vi "Min_Max_Amp (SubVI).vi"(11 "waveform":waveform(dbl)) -> (1 "AMP.":dbl, 2 "MN":dbl, 3 "MX":dbl)   [LabVIEW 2017]
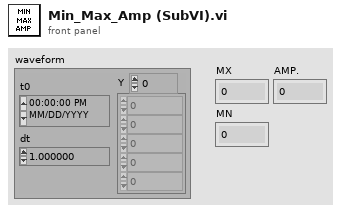
[diagram p1: front panel]
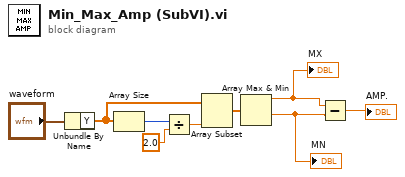
[diagram p0: block diagram]
diagram:
  n1 = Unbundle By Name("waveform") -> ("Y"=w8:dbl[])
  n2 = Array Size(array=w8) -> (size(s)=w6:i32)
  n3 = Divide(x=w6, y=2.0 ("Min Value")) -> (x/y=w5:dbl)
  n4 = Array Subset(array=w8, length=w5) -> (w9:dbl[])  [unwired: 1 in]
  n5 = Array Max & Min(array=w9) -> (max value=w3:dbl, min value=w2:dbl)  [unwired: 2 out]
  "MX" <- w3
  "MN" <- w2
  n6 = Subtract(x=w3, y=w2) -> (x-y=→"AMP.":dbl)
